vi "Get Username.vi"(8 "error in (no error)":errorcluster, 10 "User Level":enum16{"Administrator", "Engineer", "Operator"}(ring), 11 "Access in":refnum<class "Access.lvclass">) -> (0 "error out":errorcluster, 2 "Username":string[](array[string]), 3 "Access out":refnum<class "Access.lvclass">)   [LabVIEW 2021, in "Database.lvlib" / "Access.lvclass"]
uses:
  Access.lvclass
  Access.lvclass/Access.ctl
  <vilib>/addons/database/NI_Database_API.lvlib
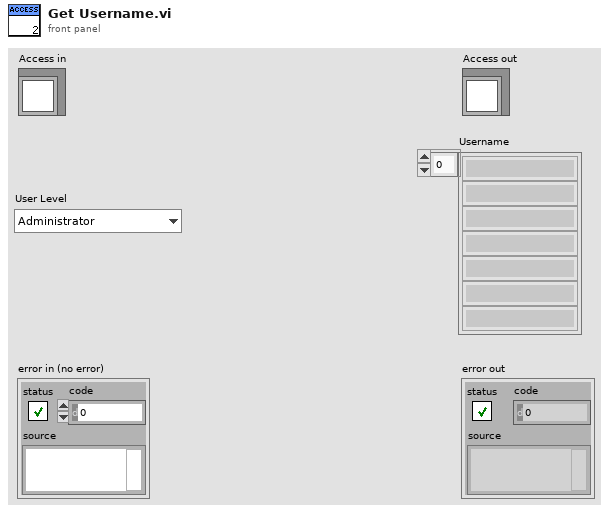
[diagram p1: front panel]
types:
  T1 = typedef "Database.lvlib/DB.lvclass/Table_info.ctl" = cluster{"Authentication":string, "Instr_Configuration":string, "Recipe":string, "Test_data":string}
  T2 = typedef "NI_Database_API.lvlib/Conn ObjectReference.ctl" = refnum<k1>
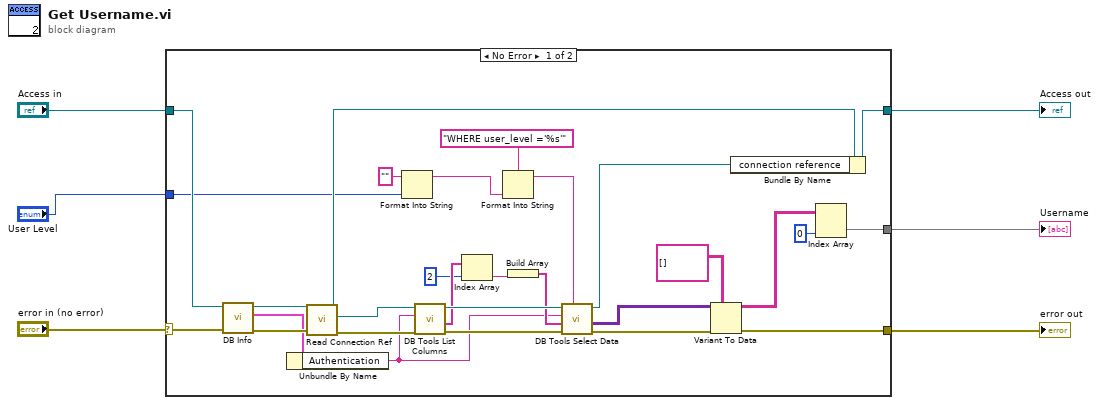
[diagram p0: block diagram]
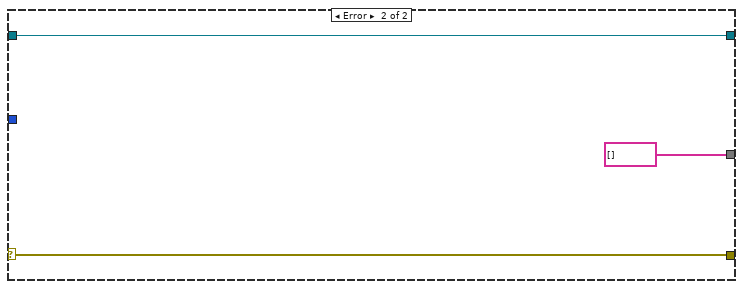
[diagram p2: hidden frame]
diagram:
  n1 = case shown="No Error" "error in (no error)" {
    selector: "error in (no error)" -> [w35 w37]
    tunnel: "Access in" -> [w34 w38]
    tunnel: [w18 w37] -> w4
    tunnel: [w16 w38] -> w3
    tunnel: [w12 string[] []] -> w2
    tunnel: "User Level" -> [w10 _]
    frame No Error {
      n2 = call-dynamic "DB Info.vi"("error in (no error)"=w35, "Access in"=w34) -> ("error out"=w32:errorcluster, "Table_info"=w21:T1, "Access out"=w33:refnum<class "Access.lvclass">)  [unwired: 6 in, 1 out]
      n3 = Unbundle By Name(w21) -> ("Authentication"=w20:string)
      n4 = call-dynamic "Read Connection Ref.vi"("error in (no error)"=w32, "Access in"=w33) -> ("error out"=w26:errorcluster, "connection reference"=w27:T2, "Access out"=w17:refnum<class "Access.lvclass">)  [unwired: 7 in]
      n5 = Format Into String(initial string="", w10) -> (resulting string=w8:string)  [unwired: 2 in, 1 out]
      n6 = call <vilib>:"DB Tools List Columns.vi"("error in (no error)"=w26, "table"=w20, "connection reference"=w27) -> ("error out"=w31:errorcluster, "columns"=w25:string[], "connection reference out"=w30:T2)  [unwired: 1 in, 1 out]
      n7 = Index Array(array=w25, index=2) -> (element=w23:string)
      n8 = Format Into String(format string="WHERE user_level ='%s'" ("condition"), w8) -> (resulting string=w7:string)  [unwired: 2 in, 1 out]
      n9 = Build Array(w23) -> (w22:string[])
      n10 = call <vilib>:"DB Tools Select Data.vi"("condition"=w7, "error in (no error)"=w31, "columns"=w22, "table"=w20, "connection reference"=w30) -> ("error out"=w29:errorcluster, "data"=w19:variant[][], "connection reference out"=w15:T2)  [unwired: 1 in]
      n11 = Variant To Data(error in=w29, type=string[][] [], Variant=w19) -> (data=w14:string[][], error out=w18:errorcluster)
      n12 = Bundle By Name(cluster=w17, "connection reference"=w15) -> (w16:refnum<class "Access.lvclass">)
      n13 = Index Array(array=w14, index (col)=0 ("disabled index (col)")) -> (element=w12:string[])  [unwired: 1 in]
    }
    frame Error {
    }
  }
  "error out" <- w4
  "Access out" <- w3
  "Username" <- w2
